vi "G4SubTemplate_Singleton_5x6x5_SetProperty.vi"(7 "Property":dbl, 11 "Error In":errorcluster) -> (15 "Error Out":errorcluster)   [LabVIEW 2020]
uses:
  <resource>/Framework/Providers/Open_GDS/ClassProviders/Provider_EndevoGOOP400/Templates/G4SubTemplate_Singleton_5x6x5/G4SubTemplate_Singleton_5x6x5.lvclass
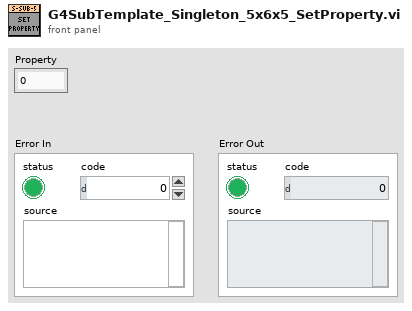
[diagram p1: front panel]
types:
  T1 = typedef "G4SubTemplate_Singleton_5x6x5.lvclass/ObjectAttributes.ctl" = cluster{"Attribute1":dbl}
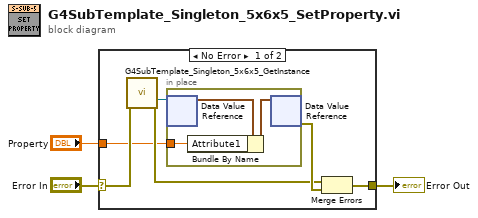
[diagram p0: block diagram]
diagram:
  n1 = case shown="No Error" "Error In" {
    selector: "Error In" -> [w9 w13]
    tunnel: [w5 w13] -> w2
    tunnel: "Property" -> [w4 _]
    frame No Error {
      n2 = call <resource>:"G4SubTemplate_Singleton_5x6x5_GetInstance.vi"("error in (no error)"=w9) -> ("DVRRefOut"=w7:refnum<data-value>, "error out"=w6:errorcluster)  [unwired: 10 in, 3 out]
      n3 = in-place {
        in-place-border: w4 -> [w12]
        n4 = in-place-dvr #1(w7) -> (w11:T1)  [unwired: 1 out]
        n5 = Bundle By Name(cluster=w11, "Attribute1"=w12) -> (w10:T1)
        n6 = in-place-dvr #1(w10) -> (w8:errorcluster)  [unwired: 1 out]
      }
      n7 = Merge Errors(w6, w8) -> (w5:errorcluster)
    }
    frame Error {
    }
  }
  "Error Out" <- w2
